vi "FP_Enable Disable Hide Control.vi"(6 "Settings":T1, 8 "Error":errorcluster, 9 "Visible":bool=TRUE, 10 "Enable":bool=TRUE, 11 "Ctl Refnum":refnum<vi>) -> (0 "Error Out":errorcluster, 1 "Disabled Out":u8, 2 "Visible Out":bool, 3 "Ctl Refnum Out":refnum<vi>, 5 "Success":bool)   [LabVIEW 2015]
uses:
  TypeDefs_Utility/ENUM_FP_Hide Show Disable.ctl
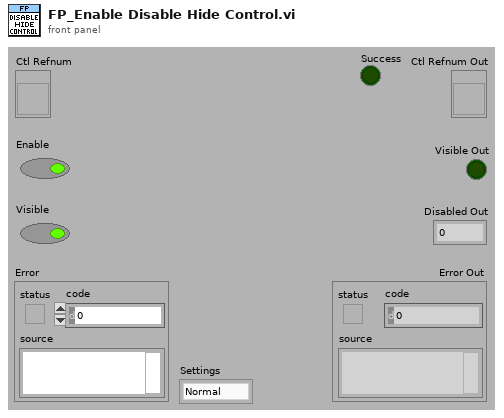
[diagram p1: front panel]
types:
  T1 = typedef "ENUM_FP_Hide Show Disable.ctl" = enum16{"Normal", "Disable", "Disable Gray", "Hide"}
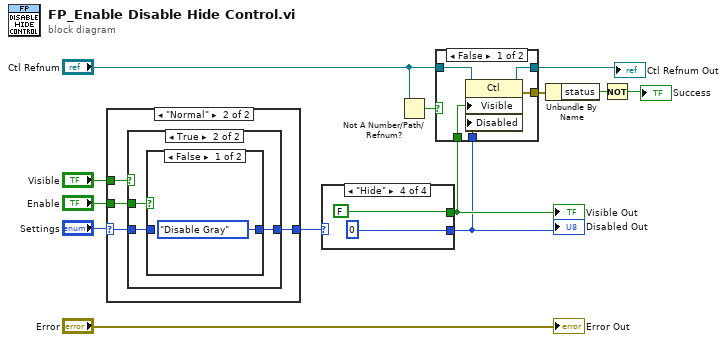
[diagram p0: block diagram]
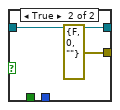
[diagram p2: hidden frame]
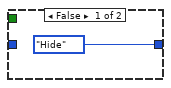
[diagram p4: hidden frame]
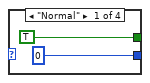
[diagram p6: hidden frame]
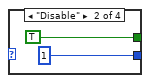
[diagram p7: hidden frame]
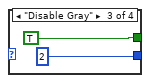
[diagram p8: hidden frame]
diagram:
  n1 = case shown="\"Normal\"" "Settings" {
    selector: "Settings" -> [w14 w18]
    tunnel: [w14 w17] -> w12
    tunnel: "Enable" -> [_ w15]
    tunnel: "Visible" -> [_ w16]
    frame "Disable".."Hide" {
    }
    frame "Normal" {
      n2 = case shown="True" w16 {
        tunnel: [ENUM_FP_Hide_Show_Disable."Hide" ("Settings") w20] -> w17
        tunnel: w18 -> [_ w21]
        tunnel: w15 -> [_ w22]
        frame False {
        }
        frame True {
          n3 = case shown="False" w22 {
            tunnel: w21 -> [_ w24]
            tunnel: [ENUM_FP_Hide_Show_Disable."Disable Gray" ("Settings") w24] -> w20
            frame False {
            }
            frame True {
            }
          }
        }
      }
    }
  }
  n4 = case shown="\"Hide\"" w12 {
    tunnel: [TRUE ("Visible") TRUE ("Visible") TRUE ("Visible") FALSE ("Visible")] -> w5
    tunnel: [u8 0 ("Disabled") u8 1 ("Disabled") u8 2 ("Disabled") u8 0 ("Disabled")] -> w4
    frame "Normal" {
    }
    frame "Disable" {
    }
    frame "Disable Gray" {
    }
    frame "Hide" {
    }
  }
  "Disabled Out" <- w4
  "Visible Out" <- w5
  n5 = Not A Number/Path/Refnum?(number/path/refnum="Ctl Refnum") -> (NaN/Path/Refnum?=w8:bool)
  n6 = case shown="False" w8 {
    tunnel: "Ctl Refnum" -> [w37 w39]
    tunnel: [w36 w39] -> w6
    tunnel: w5 -> [w35 _]
    tunnel: w4 -> [w34 _]
    tunnel: [w33 errorcluster {"status"=FALSE, "code"=0, "source"=""} ("error out")] -> w2
    frame False {
      n7 = property class="Ctl"(reference=w37, "Visible"=w35, "Disabled"=w34) -> (reference out=w36:refnum<vi>, error out=w33:errorcluster)  [unwired: 1 in]
    }
    frame True {
    }
  }
  "Ctl Refnum Out" <- w6
  n8 = Unbundle By Name(w2) -> ("status"=w3:bool)
  n9 = Not(x=w3) -> (.not. x?=→"Success":bool)
  "Error Out" <- "Error"
